vi "Cal Step.vi"(5 "Count":u8, 6 "DAC":u16[](array[numeric]), 7 "Gas Tank":u8, 9 "CalStatus":T1(ring), 10 "output cluster":T10, 11 "output cluster 3":T2 {"Current Settings"."Pump" items=["Pump 0", "Pump 1", "Pump 2", "Pump 3", "Pump 4", "Pump 5"]; "Current Settings"."Chart X axis Timescale" min=20 max=180 step=1; "Current Settings"."RunTime Mode Settings"."Exp. Gas Tank" items=["0.07", "0.031", "0.877", "1.863", "3.881", "5.790", "7.688", "6.000"]; "Current Settings"."RunTime Mode Settings"."Insp. Gas Tank" items=["0.07", "0.031", "0.877", "1.863", "3.881", "5.790", "7.688", "6.000"]; "Current Settings"."RunTime Mode Settings"."I:E Ratio" max=30 scale=0.0..7.0; "Current Settings"."RunTime Mode Settings"."Resp Rate Brpm" min=0 max=30 format="%.2f"; "Current Settings"."TE#2 Configuration"."Serial Port"."XOFF Char" format="%.0x"; "Current Settings"."TE#2 Configuration"."Serial Port"."XON Char" format="%.0x"; "Current Settings"."TE#2 Configuration"."Serial Port"."flow control" items=["None"=0, "XON/XOFF"=1, "RTS/CTS"=2, "DTR/DSR"=4]; "Current Settings"."TE#2 Configuration"."Serial Port"."stop bits" items=["1.0"=10, "1.5"=15, "2.0"=20]; "Current Settings"."TE#2 Configuration"."Serial Port"."data bits" min=5 max=8 step=1; "Current Settings"."TE#2 Configuration"."Serial Port"."baud rate" items=["75"=75, "110"=110, "134"=134, "150"=150, "300"=300, "600"=600, "1200"=1200, "1800"=1800, "2400"=2400, "4800"=4800, "7200"=7200, "9600"=9600, "14400"=14400, "19200"=19200, "28800"=28800, "38400"=38400, "56000"=56000, "57600"=57600, "115200"=115200, "128000"=128000, "230400"=230400]; "Current Settings"."TE#2 Configuration"."Serial Port"."termination char" format="%.0x"; "Current Settings"."TE#1 Configuration"."Serial Port"."XOFF Char" format="%.0x"; "Current Settings"."TE#1 Configuration"."Serial Port"."XON Char" format="%.0x"; "Current Settings"."TE#1 Configuration"."Serial Port"."flow control" items=["None"=0, "XON/XOFF"=1, "RTS/CTS"=2, "DTR/DSR"=4]; "Current Settings"."TE#1 Configuration"."Serial Port"."stop bits" items=["1.0"=10, "1.5"=15, "2.0"=20]; "Current Settings"."TE#1 Configuration"."Serial Port"."data bits" min=5 max=8 step=1; "Current Settings"."TE#1 Configuration"."Serial Port"."baud rate" items=["75"=75, "110"=110, "134"=134, "150"=150, "300"=300, "600"=600, "1200"=1200, "1800"=1800, "2400"=2400, "4800"=4800, "7200"=7200, "9600"=9600, "14400"=14400, "19200"=19200, "28800"=28800, "38400"=38400, "56000"=56000, "57600"=57600, "115200"=115200, "128000"=128000, "230400"=230400]; "Current Settings"."TE#1 Configuration"."Serial Port"."termination char" format="%.0x"; "Current Settings"."Capnometer Configuration"."Device" items=["None", "TidalWave", "LoFlow / Canary", "Capnogard"]; "Current Settings"."Capnometer Configuration"."Serial Port"."XOFF Char" format="%.0x"; "Current Settings"."Capnometer Configuration"."Serial Port"."XON Char" format="%.0x"; "Current Settings"."Capnometer Configuration"."Serial Port"."flow control" items=["None"=0, "XON/XOFF"=1, "RTS/CTS"=2, "DTR/DSR"=4]; "Current Settings"."Capnometer Configuration"."Serial Port"."stop bits" items=["1.0"=10, "1.5"=15, "2.0"=20]; "Current Settings"."Capnometer Configuration"."Serial Port"."data bits" min=5 max=8 step=1; "Current Settings"."Capnometer Configuration"."Serial Port"."baud rate" items=["75"=75, "110"=110, "134"=134, "150"=150, "300"=300, "600"=600, "1200"=1200, "1800"=1800, "2400"=2400, "4800"=4800, "7200"=7200, "9600"=9600, "14400"=14400, "19200"=19200, "28800"=28800, "38400"=38400, "56000"=56000, "57600"=57600, "115200"=115200, "128000"=128000, "230400"=230400]; "Current Settings"."Capnometer Configuration"."Serial Port"."termination char" format="%.0x"; "Current Settings"."DAQx Settings"."Analog Output Settings (Volts)" format="%#.3g"; "Current Settings"."DAQx Settings"."Duty Cycle" min=10.0 max=90.0 format="%.1g"; "Current Settings"."DAQx Settings"."Frequency" min=20.0 max=200.0; "Current Settings"."DataLogging Settings"."Data File Duration (Minutes)" min=2 max=200 format="%#.2g"; "Current Settings"."Calibration Settings"."Tolerance #2" min=2 max=4096; "Current Settings"."Calibration Settings"."Cal. Average" min=2 max=4096; "Current Settings"."Test Settings"."Test Sensor ID" items=["(select)", "RB", "YC", "", "Other"]}) -> (1 "NewCalStatus":T1(ring), 2 "New Count":u8)   [LabVIEW 2016]
uses:
  Controls/Cal Refs.ctl
  Controls/DAQ Needed.ctl
  Controls/Processed Variables.ctl
  Controls/AirPump Controls.ctl
  Controls/IE Ratio knob.ctl
  Controls/UI Settings.ctl
  Controls/Aux CO2 Control.ctl
  Controls/Serial Visa Control.ctl
  Controls/Aux CO2 Selector.ctl
  Controls/Aux TE Control.ctl
  Controls/Queues And Others.ctl
  <vilib>/Analysis/baseanly.llb/Mean (DBL).vi
  Miscellaneous/Globals.vi
  <vilib>/Analysis/NI_AALBase.lvlib
panel:
  # "Note: Setting Brpm to zero will\ndisable Insp / Exp digital output."
  # "mmHg"
  # "pts"
  # "tolerance"
  # "AN5 (Temp 1)"
  # "AN6 (Temp 2)"
  # "AN7 (Temp 3)"
  # "AN8 (T FET)"
  # "AN0 (T POT)"
  # "Tref (Set Pt))"
  # "(Spare)"
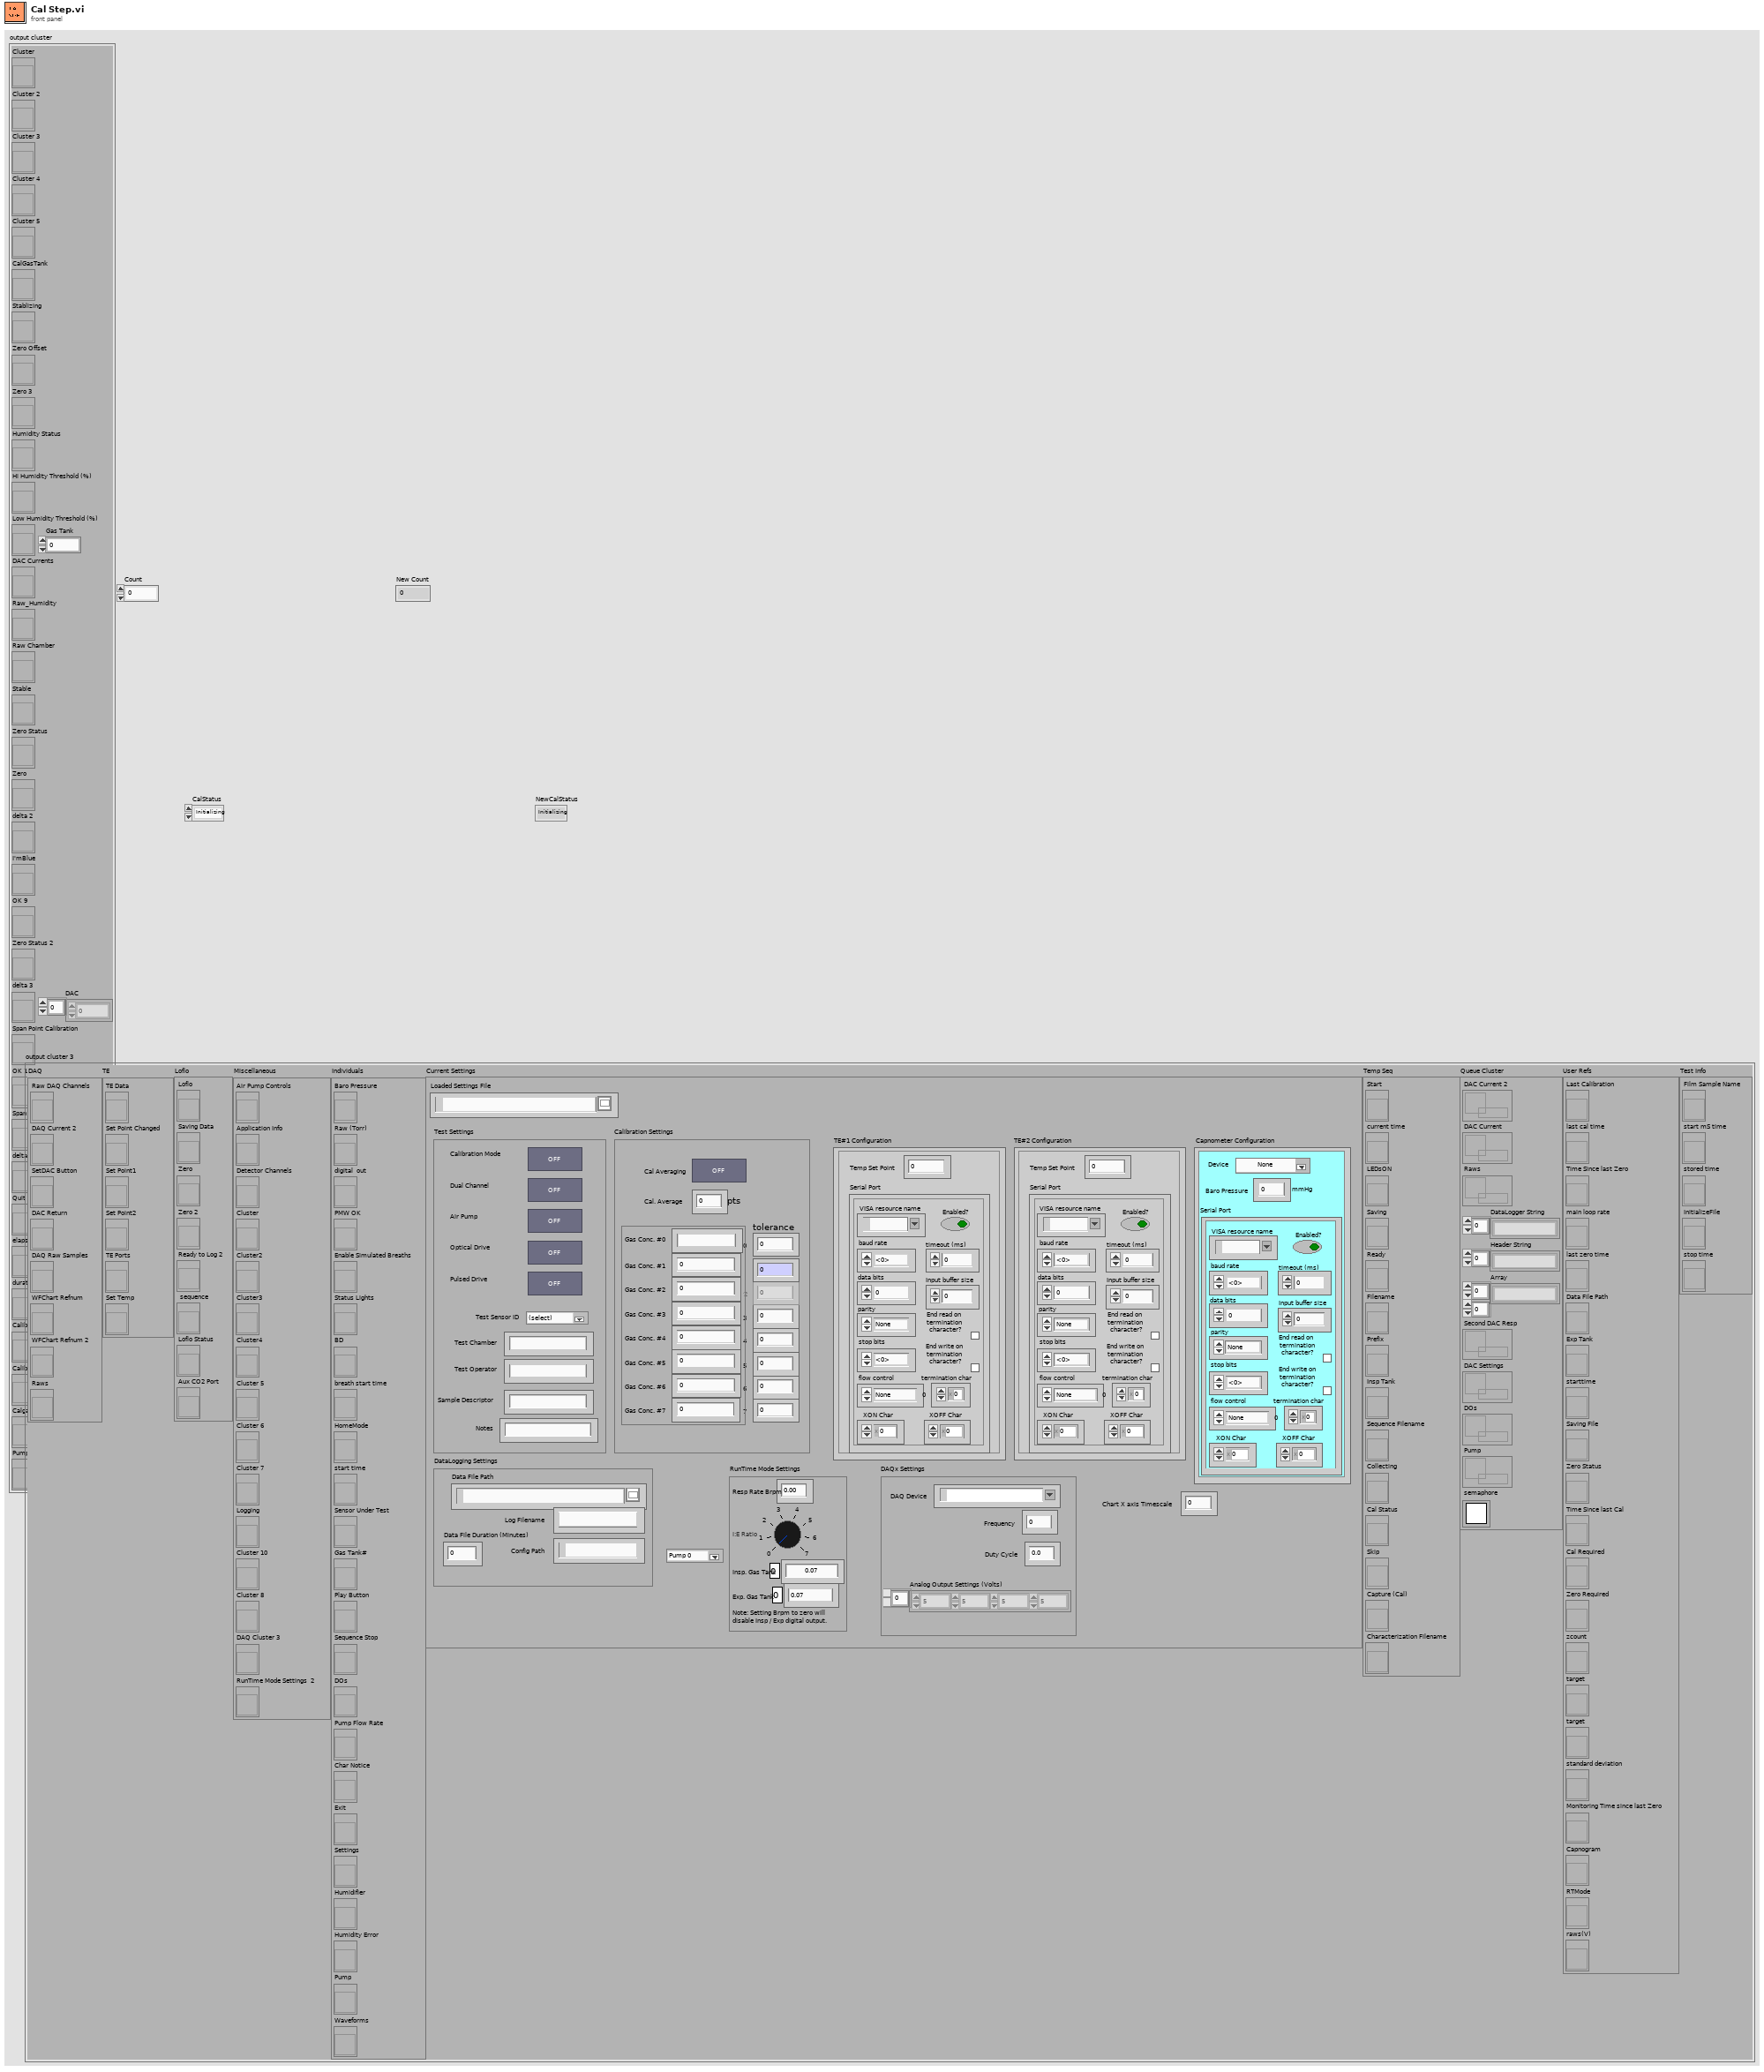
[diagram p1: front panel]
types:
  T1 = enum32{"Initializing", "Enter CO2 Value", "Enter Calibration Code", "Reading Calibration Data", "Stablizing", "Calculating Target Voltages", "Setting Zero Point", "Setting High Point", "Setting Span Point", "Calculating Gain & Offset", "Storing Calibration Coefficients", "Calibration Complete"}
  T2 = typedef "DAQ Needed.ctl" = cluster{"DAQ":cluster{"Raw DAQ Channels":refnum<vi>, "DAQ Current 2":refnum<vi>, "SetDAC Button":refnum<vi>, "DAC Return":refnum<vi>, "DAQ Raw Samples":refnum<vi>, "WFChart Refnum":refnum<vi>, "WFChart Refnum 2":refnum<vi>, "Raws":refnum<vi>}, "TE":cluster{"TE Data":refnum<vi>, "Set Point Changed":refnum<vi>, "Set Point1":refnum<vi>, "Set Point2":refnum<vi>, "TE Ports":refnum<vi>, "Set Temp":refnum<vi>}, "Loflo":cluster{"Loflo":refnum<vi>, "Saving Data":refnum<vi>, "Zero":refnum<vi>, "Zero 2":refnum<vi>, "Ready to Log 2":refnum<vi>, " sequence":refnum<vi>, "Loflo Status ":refnum<vi>, "Aux CO2 Port":refnum<vi>}, "Miscellaneous":cluster{"Air Pump Controls":refnum<vi>, "Application Info":refnum<vi>, "Detector Channels ":refnum<vi>, "Cluster":refnum<vi>, "Cluster2":refnum<vi>, "Cluster3":refnum<vi>, "Cluster4":refnum<vi>, "Cluster 5":refnum<vi>, "Cluster 6":refnum<vi>, "Cluster 7":refnum<vi>, "Logging":refnum<vi>, "Cluster 10":refnum<vi>, "Cluster 8":refnum<vi>, "DAQ Cluster 3":refnum<vi>, "RunTime Mode Settings  2":refnum<vi>}, "Individuals":cluster{"Baro Pressure":refnum<vi>, "Raw (Torr)":refnum<vi>, "digital  out":refnum<vi>, "PMW OK":refnum<vi>, "Enable Simulated Breaths":refnum<vi>, "Status Lights":refnum<vi>, "BD":refnum<vi>, "breath start time":refnum<vi>, "HomeMode":refnum<vi>, "start time":refnum<vi>, "Sensor Under Test":refnum<vi>, "Gas Tank#":refnum<vi>, "Play Button":refnum<vi>, "Sequence Stop":refnum<vi>, "DOs":refnum<vi>, "Pump Flow Rate":refnum<vi>, "Char Notice":refnum<vi>, "Exit":refnum<vi>, "Settings":refnum<vi>, "Humidifier":refnum<vi>, "Humidity Error":refnum<vi>, "Pump":refnum<vi>, "Waveforms":refnum<vi>}, "Current Settings":T3, "Temp Seq":cluster{"Start":refnum<vi>, "current time":refnum<vi>, "LEDsON":refnum<vi>, "Saving":refnum<vi>, "Ready":refnum<vi>, "Filename":refnum<vi>, "Prefix":refnum<vi>, "Insp Tank":refnum<vi>, "Sequence Filename":refnum<vi>, "Collecting":refnum<vi>, "Cal Status":refnum<vi>, "Skip":refnum<vi>, "Capture (Cal)":refnum<vi>, "Characterization Filename":refnum<vi>}, "Queue Cluster":T8, "User Refs":cluster{"Last Calibration":refnum<vi>, "last cal time":refnum<vi>, "Time Since last Zero":refnum<vi>, "main loop rate":refnum<vi>, "last zero time":refnum<vi>, "Data File Path":refnum<vi>, "Exp Tank":refnum<vi>, "starttime":refnum<vi>, "Saving File":refnum<vi>, "Zero Status":refnum<vi>, "Time Since last Cal":refnum<vi>, "Cal Required":refnum<vi>, "Zero Required":refnum<vi>, "zcount":refnum<vi>, "target":refnum<vi>, "target":refnum<vi>, "standard deviation":refnum<vi>, "Monitoring Time since last Zero":refnum<vi>, "Capnogram":refnum<vi>, "RTMode":refnum<vi>, "raws(V)":refnum<vi>}, "Test Info":cluster{"Film Sample Name":refnum<vi>, "start mS time":refnum<vi>, "stored time":refnum<vi>, "InitializeFile":refnum<vi>, "stop time":refnum<vi>}}
  T3 = typedef "UI Settings.ctl" = cluster{"Loaded Settings File":path, "Test Settings":cluster{"Dual Channel":bool, "Air Pump":bool, "Optical Drive":bool, "Pulsed Drive":bool, "Calibration Mode":bool, "Test Sensor ID":u16, "Test Chamber":string, "Test Operator":string, "Sample Descriptor":string, "Notes":string}, "Calibration Settings":cluster{"Cal. Average":u16, "Cal Averaging":bool, "Tolerance #0":sgl, "Tolerance #7":sgl, "Tolerance #6":sgl, "Tolerance #5":sgl, "Tolerance #4":sgl, "Tolerance #3":sgl, "Tolerance #2":sgl, "Tolerance #1":sgl, "Gas Tank Settings":cluster{"Gas Conc. #0":string, "Gas Conc. #1":sgl, "Gas Conc. #2":sgl, "Gas Conc. #3":sgl, "Gas Conc. #4":sgl, "Gas Conc. #5":sgl, "Gas Conc. #6":sgl, "Gas Conc. #7":sgl}}, "DataLogging Settings":cluster{"Data File Path":path, "Data File Duration (Minutes)":sgl, "Log Filename":string, "Config Path":path}, "DAQx Settings":cluster{"DAQ Device":tag, "Frequency":dbl, "Duty Cycle":dbl, "Analog Output Settings (Volts)":sgl[]}, "Capnometer Configuration":T4, "TE#1 Configuration":T7, "TE#2 Configuration":T7, "RunTime Mode Settings ":cluster{"Resp Rate Brpm ":sgl, "I:E Ratio":u8, "Insp. Gas Tank":u16, "Exp. Gas Tank":u16}, "Chart X axis Timescale":u16, "Pump":u16}
  T4 = typedef "Aux CO2 Control.ctl" = cluster{"Serial Port":T5, "Baro Pressure":u32, "Device":T6}
  T5 = typedef "Serial Visa Control.ctl" = cluster{"termination char":u8, "End read on termination character?":bool, "Enabled?":bool, "VISA resource name":refnum<visa-resource-name>, "baud rate":u32, "data bits":u16, "parity":enum16{"None", "Odd", "Even", "Mark", "Space"}, "stop bits":u16, "flow control":u16, "timeout (ms)":u32, "Input buffer size":u32, "End write on termination character?":bool, "XON Char":u8, "XOFF Char":u8}
  T6 = typedef "Aux CO2 Selector.ctl" = u16
  T7 = typedef "Aux TE Control.ctl" = cluster{"Temp Set Point":sgl, "Serial Port":T5}
  T8 = typedef "Queues And Others.ctl" = cluster{"DAC Current 2":refnum<queue>, "DAC Current":refnum<queue>, "Raws":refnum<queue>, "DataLogger String":string[], "Header String":string[], "Array":string[][], "Second DAC Resp":refnum<queue>, "DAC Settings":refnum<queue>, "DOs":refnum<queue>, "Pump":refnum<queue>, "semaphore":T9}
  T9 = typedef "Semaphore RefNum" = refnum<k1>
  T10 = typedef "Cal Refs.ctl" = cluster{"Cluster":refnum<vi>, "Cluster 2":refnum<vi>, "Cluster 3":refnum<vi>, "Cluster 4":refnum<vi>, "Cluster 5":refnum<vi>, "CalGasTank":refnum<vi>, "Stablizing":refnum<vi>, "Zero Offset":refnum<vi>, "Zero 3":refnum<vi>, "Humidity Status":refnum<vi>, "Hi Humidity Threshold (%)":refnum<vi>, "Low Humidity Threshold (%)":refnum<vi>, "DAC Currents":refnum<vi>, "Raw_Humidity":refnum<vi>, "Raw Chamber":refnum<vi>, "Stable":refnum<vi>, "Zero Status":refnum<vi>, "Zero":refnum<vi>, "delta 2":refnum<vi>, "I'mBlue":refnum<vi>, "OK 9":refnum<vi>, "Zero Status 2":refnum<vi>, "delta 3":refnum<vi>, "Span Point Calibration":refnum<vi>, "OK 10":refnum<vi>, "Span Good":refnum<vi>, "delta":refnum<vi>, "Quit":refnum<vi>, "elapsed time":refnum<vi>, "duration":refnum<vi>, "Calibration Complete -":refnum<vi>, "Calibration Complete":refnum<vi>, "Calgas":refnum<vi>, "Pump Settings":refnum<vi>}
  T11 = cluster{"Tcal_Chamber":dbl, "Tcal_PCB":dbl, "Tcal_Film":dbl, "Tcal_Humidity":dbl, "Tcal_Det":dbl[], "Cal Gas":dbl, "Reference":dbl}
  T12 = cluster{"CalFile Selected":path, "TYPE":string, "DATE":string, "C0FC2V":dbl[], "C6FC2V":dbl[], "V_0d(target)":dbl[], "V_6d(target)":dbl[], "V_span(target)":dbl[], "CHANNEL":string[], "Status":bool[], "BlueLED 2":bool[], "C2V":u8[], "A":dbl[], "B":dbl[], "C":dbl[], "D":dbl[], "V2C":u8[], "A'":dbl[], "B'":dbl[], "C'":dbl[], "D'":dbl[]}
  T13 = cluster{"CHANNEL 2":string[], "BlueLED":bool[], "V_RA(5mA)":dbl[], "V_RA(15mA)":dbl[], "mI":dbl[], "DAC scale":dbl[]}
  T14 = cluster{"V_0d(ImA)\nActual":dbl[], "V_6d(ImA)\nActual":dbl[], "V_span(ImA)":dbl[], "V_0(adjust)\ncal offsets":dbl[], "V_span(adjust)":dbl[], "Gain(adjust)":dbl[]}
  T15 = typedef "Calibration Coefficients.ctl" = cluster{"CalFile Used":path, "TYPE":string, "DATE":string, "Humidity":sgl, "Chamber Temp":dbl, "CO2_calgas":dbl, "V_(RA,5mA)":dbl, "V_(RA,15mA)":dbl, "mI":dbl, "V_0d_ImA (actual)":dbl, "V_6d_ImA (actual)":dbl, "I_span":dbl, "DAC":u16, "A":dbl, "B":dbl, "C":dbl, "D":dbl, "V6d":dbl, "A'":dbl, "B'":dbl, "C'":dbl, "D'":dbl, "V0d":dbl, "CalDate":string, "CalTime":string, "duration":dbl, "Detector Channel":string, "a2":dbl, "a3":dbl, "a4":dbl, "a5":dbl, "b2":dbl, "c2":dbl, "b3":dbl, "c3":dbl, "b4":dbl, "c4":dbl, "b5":dbl, "c5":dbl, "a7":dbl, "a8":dbl, "a9":dbl, "a10":dbl, "b7":dbl, "b8":dbl, "b9":dbl, "b10":dbl, "c7":dbl, "c8":dbl, "c9":dbl, "c10":dbl, "cal_offs_adj":dbl, "cal_gain_adj":dbl, "C6d":dbl, "C0d":dbl, "Cal_currernt":dbl, "C2V":u16, "V2C":u16, "Zero Date":string, "Zero Time":string, "Number of Zeroes":u16, "V_(()d, average)":dbl, "V_offs ":dbl, "G_adj":dbl, "Pump Flow Rate":u16, "Zero Required? ":bool, "Calibrate Required?":bool, "cal_utc":dbl, "zero_utc":dbl, "Elapsed Time":dbl, "PCB":string, "m0":dbl, "b0":dbl}
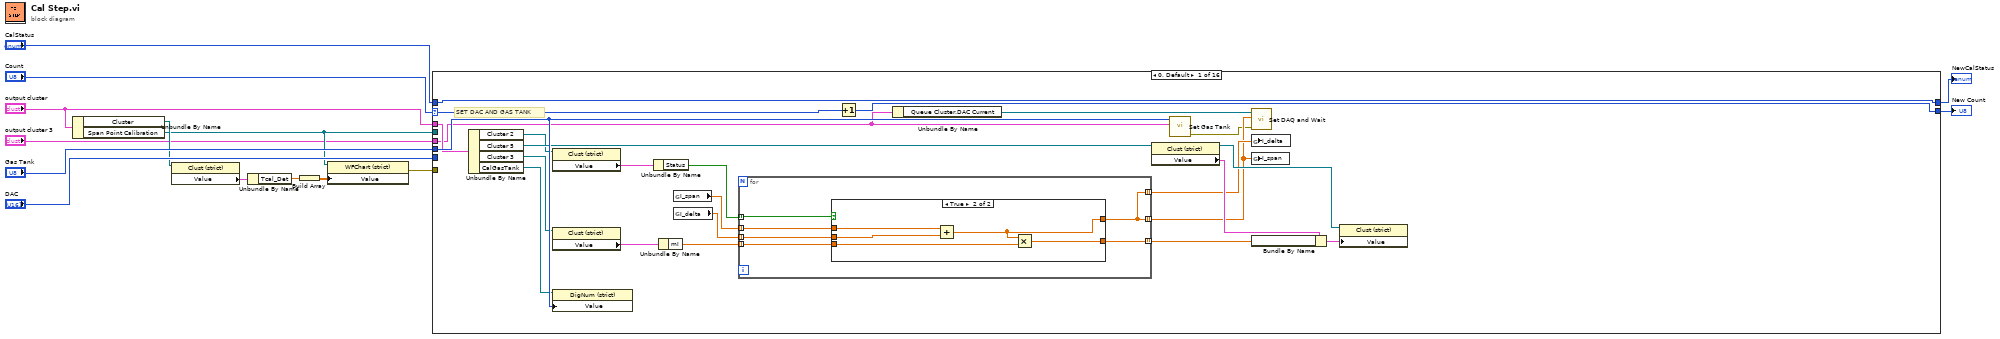
[diagram p0: block diagram]
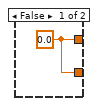
[diagram p2: hidden frame]
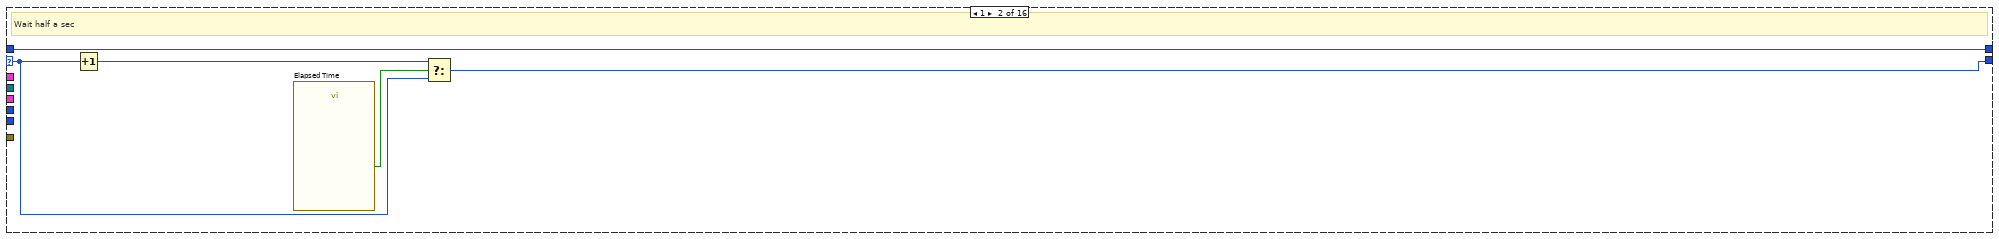
[diagram p3: hidden frame]
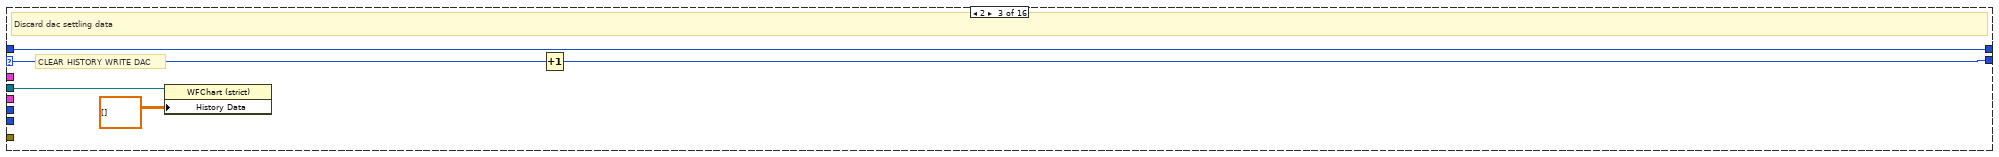
[diagram p4: hidden frame]
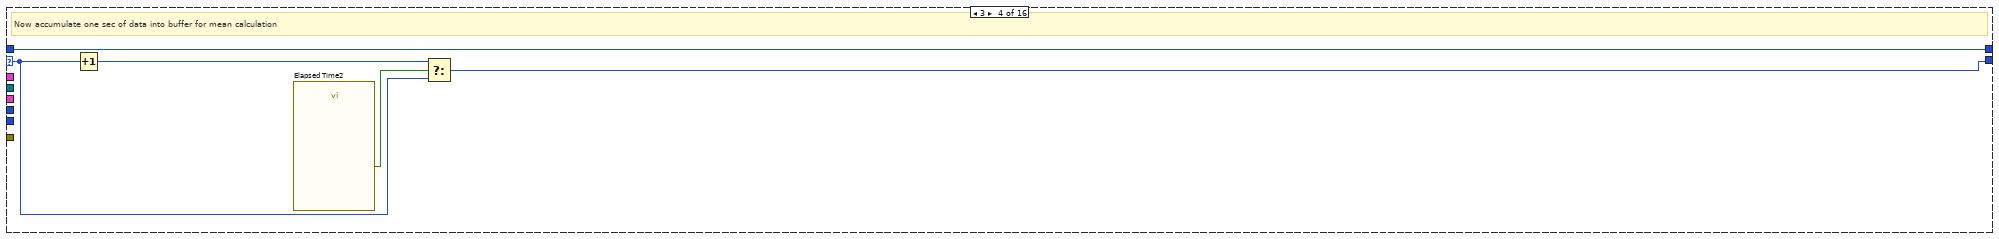
[diagram p5: hidden frame]
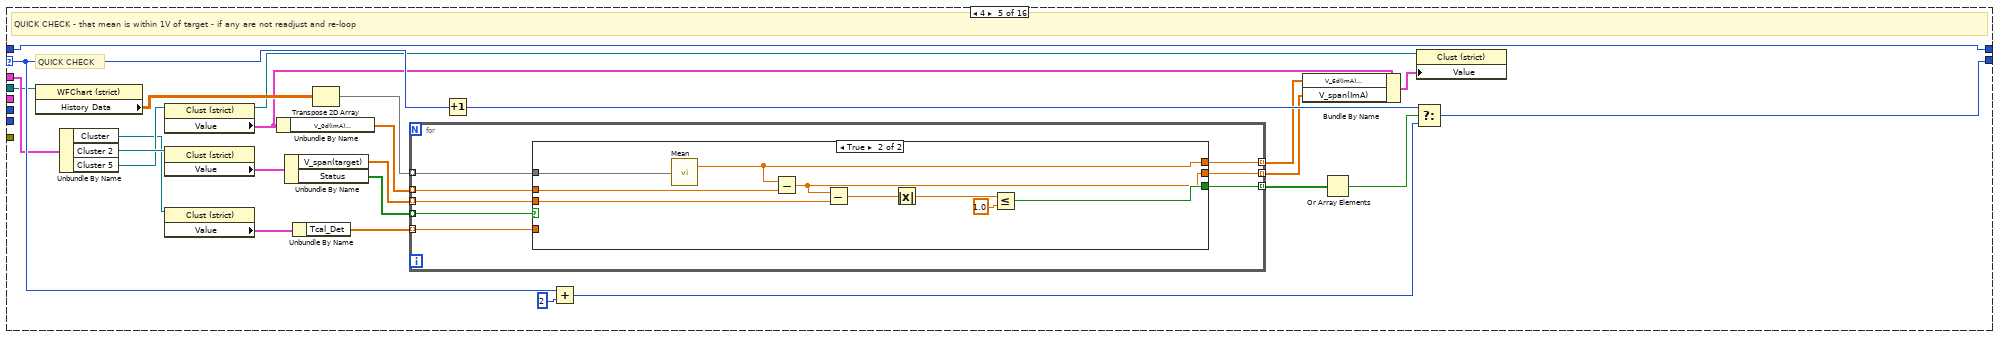
[diagram p6: hidden frame]
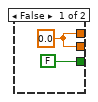
[diagram p7: hidden frame]
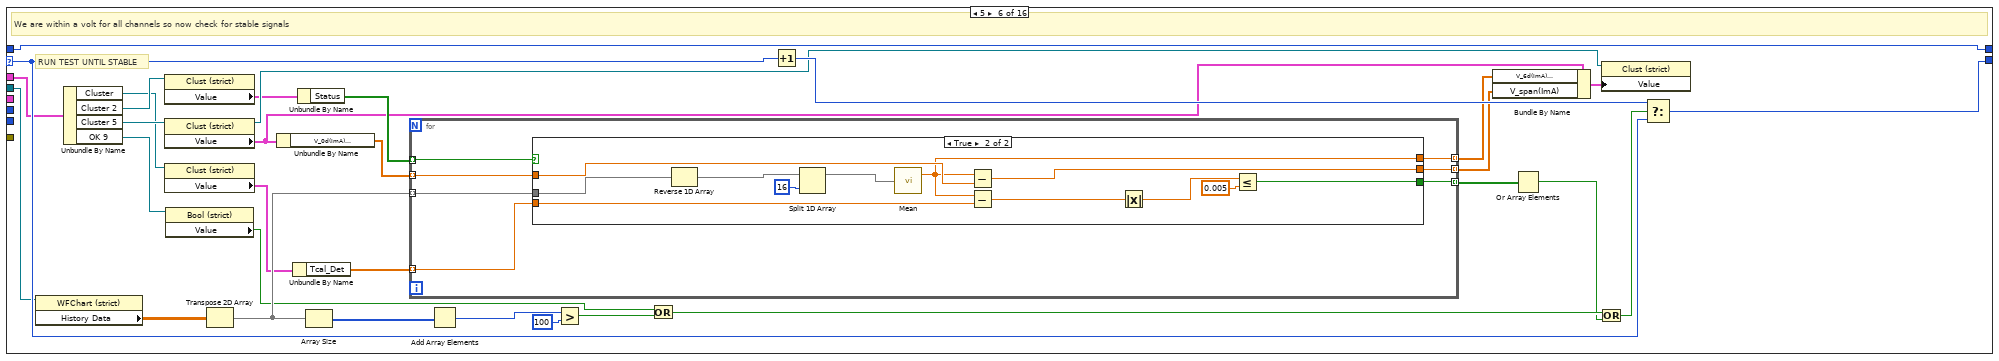
[diagram p8: hidden frame]
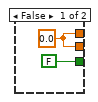
[diagram p9: hidden frame]
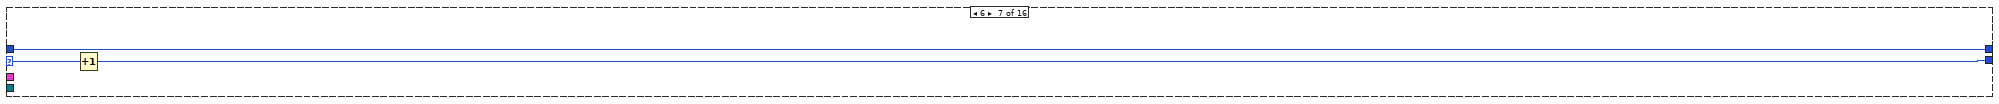
[diagram p10: hidden frame]
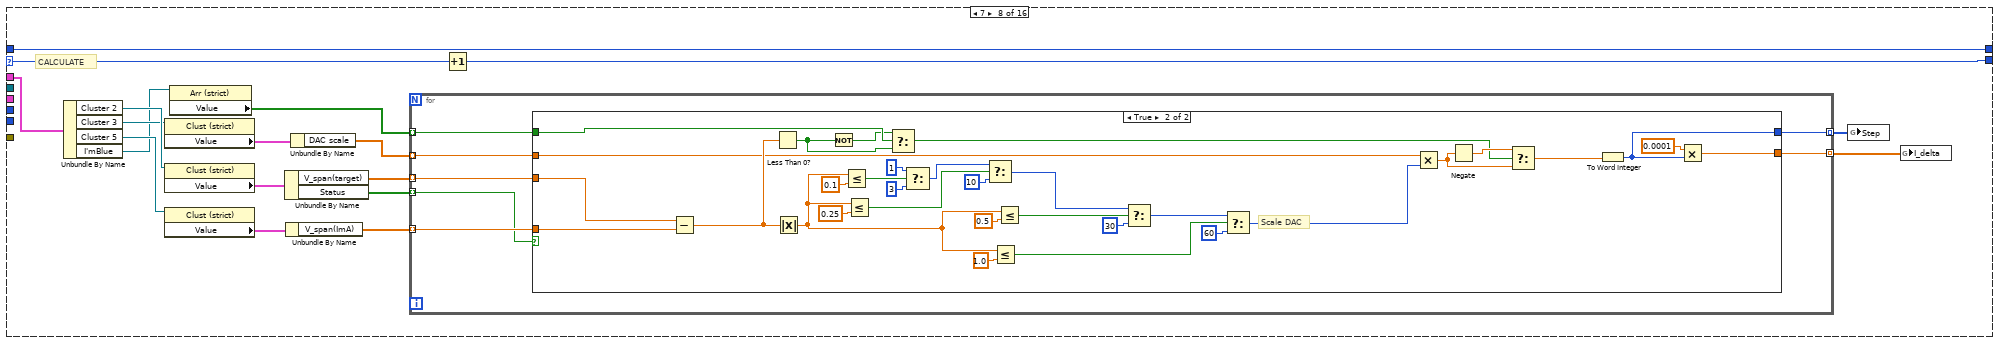
[diagram p11: hidden frame]
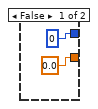
[diagram p12: hidden frame]
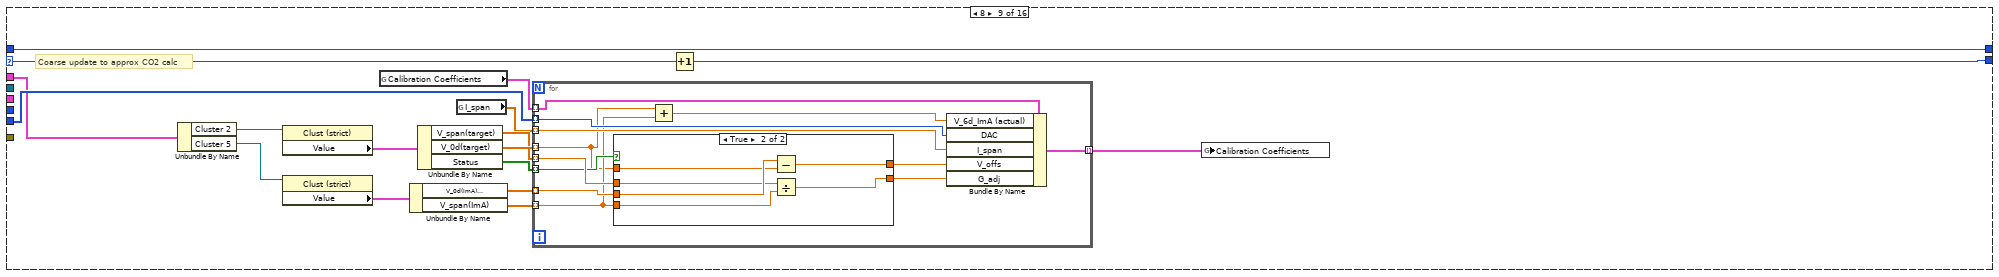
[diagram p13: hidden frame]
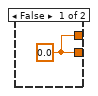
[diagram p14: hidden frame]
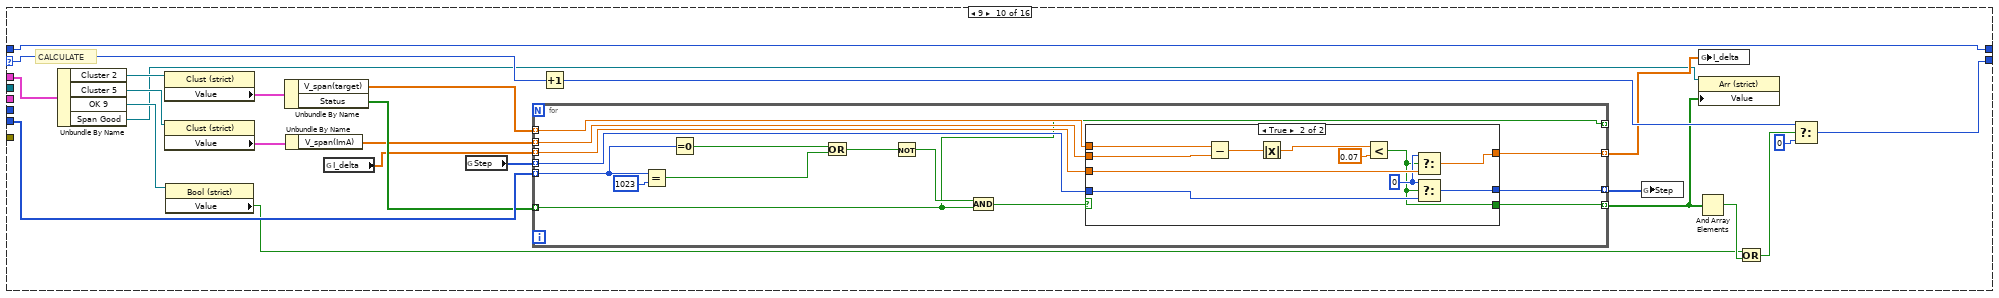
[diagram p15: hidden frame]
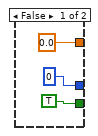
[diagram p16: hidden frame]
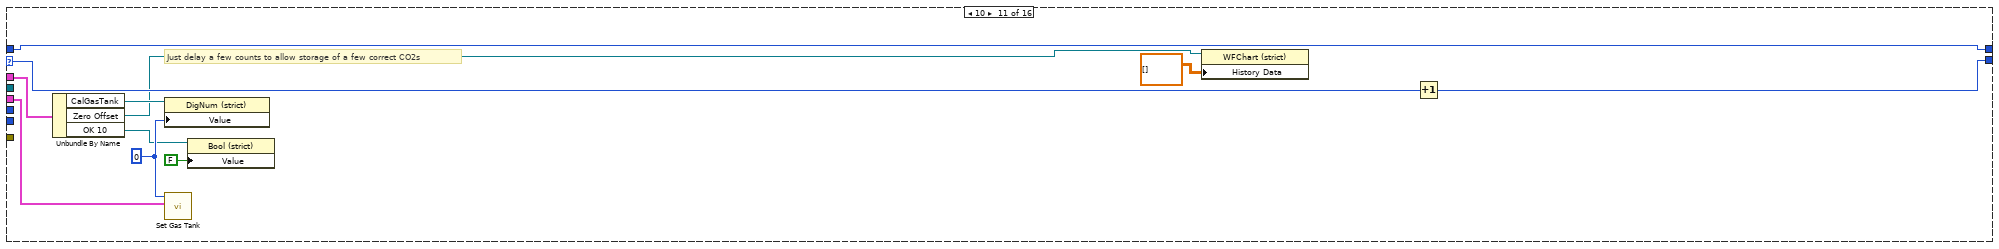
[diagram p17: hidden frame]
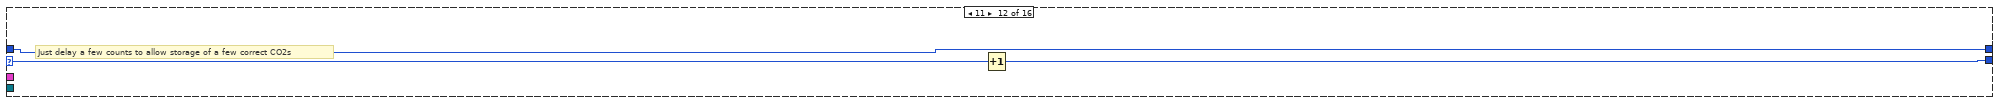
[diagram p18: hidden frame]
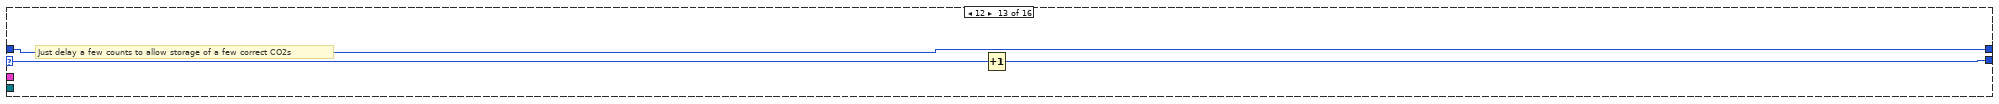
[diagram p19: hidden frame]
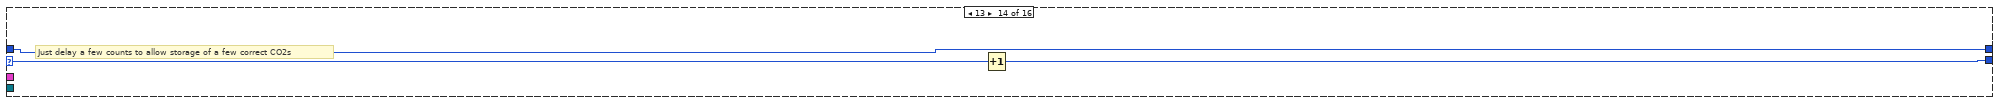
[diagram p20: hidden frame]
diagram:
  n1 = Unbundle By Name("output cluster") -> ("Cluster"=w9:refnum<vi>, "Span Point Calibration"=w6:refnum<vi>)
  n2 = property class="Clust (strict)"(reference=w9) -> ("Value"=w12:T11)  [unwired: 1 in, 2 out]
  n3 = Unbundle By Name(w12) -> ("Tcal_Det"=w11:dbl[])
  n4 = Build Array(w11) -> (w8:dbl[][])
  n5 = property class="WFChart (strict)"(reference=w6, "Value"=w8) -> (error out=w7:errorcluster)  [unwired: 1 in, 1 out]
  n6 = case shown="0, Default" "Count" {
    selector: "Count" -> [w37 w52 w60 w63 w88 w137 w165 w183 w241 w279 w324 w327 w330 w333 w336 _]
    tunnel: [w36 w54 w59 w62 w89 w138 w164 w181 w240 w280 w323 w326 w329 w332 w335 0 ("Step")] -> w1
    tunnel: "CalStatus" -> [w38 w55 w58 w65 w91 w141 w163 w182 w239 w284 w322 w325 w328 w331 w334 w339]
    tunnel: [w38 w55 w58 w65 w91 w141 w163 w182 w239 w284 w322 w325 w328 w331 w334 w337] -> w3
    tunnel: "Gas Tank" -> [w33 _ _ _ _ _ _ _ _ _ _ _ _ _ _ _]
    tunnel: "DAC" -> [_ _ _ _ _ _ _ _ w238 w276 _ _ _ _ _ _]
    tunnel: "output cluster 3" -> [w21 _ _ _ _ _ _ _ _ _ w315 _ _ _ _ _]
    tunnel: "output cluster" -> [w28 _ _ _ w77 w123 _ w180 w235 w274 w314 _ _ _ _ _]
    tunnel: w6 -> [_ _ w56 _ w66 w113 _ _ _ _ _ _ _ _ _ _]
    tunnel: w7 -> [_ _ _ _ _ _ _ _ _ _ _ _ _ _ _ _]
    frame 0, Default {
      # "SET DAC AND GAS TANK"
      n7 = Unbundle By Name(w28) -> ("Cluster 2"=w24:refnum<vi>, "Cluster 5"=w25:refnum<vi>, "Cluster 3"=w26:refnum<vi>, "CalGasTank"=w27:refnum<vi>)
      n8 = property class="Clust (strict)"(reference=w24) -> ("Value"=w23:T12)  [unwired: 1 in, 2 out]
      n9 = property class="Clust (strict)"(reference=w26) -> ("Value"=w35:T13)  [unwired: 1 in, 2 out]
      n10 = property class="DigNum (strict)"(reference=w27, "Value"=w33) -> ()  [unwired: 1 in, 2 out]
      n11 = Unbundle By Name(w23) -> ("Status"=w22:bool[])
      n12 = Unbundle By Name(w35) -> ("mI"=w34:dbl[])
      n13 = global read "Globals.vi" "I_span"() -> (w20:dbl[])
      n14 = global read "Globals.vi" "I_delta"() -> (w18:dbl[])
      n15 = for {
        tunnel: w34 -> [w42] mode=indexing
        tunnel: [w41] -> w29 mode=indexing
        tunnel: w20 -> [w44] mode=indexing
        tunnel: w18 -> [w43] mode=indexing
        tunnel: [w40] -> w19 mode=indexing
        tunnel: [w40] -> w16 mode=indexing
        tunnel: w22 -> [w39] mode=indexing
        n16 = case shown="True" w39 {
          tunnel: w44 -> [_ w50]
          tunnel: w43 -> [_ w49]
          tunnel: w42 -> [_ w48]
          tunnel: [w45 w47] -> w41
          tunnel: [w45 w46] -> w40
          frame False {
            w45 = 0.0
          }
          frame True {
            n17 = Add(x=w50, y=w49) -> (x+y=w46:dbl)
            n18 = Multiply(x=w46, y=w48) -> (x*y=w47:dbl)
          }
        }
      }
      n19 = Increment(x=w37) -> (x+1=w36:u8)
      n20 = Unbundle By Name(w21) -> ("Queue Cluster.DAC Current"=w17:refnum<queue>)
      n21 = property class="Clust (strict)"(reference=w25) -> (reference out=w32:refnum<vi>, "Value"=w31:T14)  [unwired: 1 in, 1 out]
      n22 = call "Set Gas Tank.vi"("input cluster"=w21, "Gas Tank"=w33) -> ("error out"=w15:errorcluster)  [unwired: 8 in, 1 out]
      n23 = call "Set DAQ and Wait.vi"("error in (no error)"=w15, "Array"=w16, "Queue in"=w17) -> ()  [unwired: 9 in]
      n24 = global write "Globals.vi" "I_delta"(w19) -> ()
      n25 = global write "Globals.vi" "I_span"(w16) -> ()
      n26 = Bundle By Name(cluster=w31, "V_0d(ImA)\nActual"=w29) -> (w30:T14)
      n27 = property class="Clust (strict)"(reference=w32, "Value"=w30) -> ()  [unwired: 1 in, 2 out]
    }
    frame 1 {
      # "Wait half a sec"
      n28 = Increment(x=w52) -> (x+1=w53:u8)
      n29 = call "Elapsed Time"() -> ("Time has Elapsed"=w51:bool)  [unwired: 12 in, 7 out]
      n30 = Select(t=w53, s=w51, f=w52) -> (s? t:f=w54:u8)
    }
    frame 2 {
      # "CLEAR HISTORY WRITE DAC"
      # "Discard dac settling data"
      n31 = property on="Property Node" class="WFChart (strict)"(reference=w56, "History Data"=dbl[][] []) -> ()  [unwired: 1 in, 2 out]
      n32 = Increment(x=w60) -> (x+1=w59:u8)
    }
    frame 3 {
      # "Now accumulate one sec of data into buffer for mean calculation"
      n33 = Increment(x=w63) -> (x+1=w64:u8)
      n34 = call "Elapsed Time2"() -> ("Time has Elapsed"=w61:bool)  [unwired: 12 in, 7 out]
      n35 = Select(t=w64, s=w61, f=w63) -> (s? t:f=w62:u8)
    }
    frame 4 {
      # "QUICK CHECK"
      # "QUICK CHECK - that mean is within 1V of target - if any are not readjust and re-loop"
      n36 = property on="Property Node" class="WFChart (strict)"(reference=w66) -> ("History Data"=w83:dbl[][])  [unwired: 1 in, 2 out]
      n37 = Unbundle By Name(w77) -> ("Cluster"=w71:refnum<vi>, "Cluster 2"=w76:refnum<vi>, "Cluster 5"=w73:refnum<vi>)
      n38 = property class="Clust (strict)"(reference=w73) -> (reference out=w81:refnum<vi>, "Value"=w68:T14)  [unwired: 1 in, 1 out]
      n39 = property class="Clust (strict)"(reference=w76) -> ("Value"=w75:T12)  [unwired: 1 in, 2 out]
      n40 = property class="Clust (strict)"(reference=w71) -> ("Value"=w72:T11)  [unwired: 1 in, 2 out]
      n41 = Unbundle By Name(w68) -> ("V_0d(ImA)\nActual"=w67:dbl[])
      n42 = Unbundle By Name(w75) -> ("V_span(target)"=w69:dbl[], "Status"=w74:bool[])
      n43 = Unbundle By Name(w72) -> ("Tcal_Det"=w70:dbl[])
      n44 = Transpose 2D Array(2D array=w83) -> (transposed array=w82:dbl[][])
      n45 = for {
        tunnel: w82 -> [w97] mode=indexing
        tunnel: [w99] -> w85 mode=indexing
        tunnel: w70 -> [w98] mode=indexing
        tunnel: [w95] -> w78 mode=indexing
        tunnel: [w96] -> w79 mode=indexing
        tunnel: w67 -> [w94] mode=indexing
        tunnel: w74 -> [w93] mode=indexing
        tunnel: w69 -> [w92] mode=indexing
        n46 = case shown="True" w93 {
          tunnel: [FALSE w110] -> w99
          tunnel: w98 -> [_ _]
          tunnel: w97 -> [_ w109]
          tunnel: [w101 w108] -> w96
          tunnel: [w101 w102] -> w95
          tunnel: w94 -> [_ w107]
          tunnel: w92 -> [_ w103]
          frame False {
            w101 = 0.0
          }
          frame True {
            n47 = call-poly <vilib>:"Mean.vi"("X"=w109) -> ("mean"=w108:dbl)  [unwired: 1 out]
            n48 = Subtract(x=w108, y=w107) -> (x-y=w102:dbl)
            n49 = Subtract(x=w102, y=w103) -> (x-y=w104:dbl)
            n50 = Absolute Value(x=w104) -> (abs(x)=w105:dbl)
            n51 = Less Or Equal?(x=w105, y=1.0) -> (x <= y?=w110:bool)
          }
        }
      }
      n52 = Increment(x=w88) -> (x+1=w90:u8)
      n53 = Add(x=w88, y=2) -> (x+y=w86:i32)
      n54 = Bundle By Name(cluster=w68, "V_6d(ImA)\nActual"=w79, "V_span(ImA)"=w78) -> (w80:T14)
      n55 = Or Array Elements(Boolean array=w85) -> (logical OR=w84:bool)
      n56 = Select(t=w90, s=w84, f=w86) -> (s? t:f=w89:i32)
      n57 = property class="Clust (strict)"(reference=w81, "Value"=w80) -> ()  [unwired: 1 in, 2 out]
    }
    frame 5 {
      # "RUN TEST UNTIL STABLE"
      # "We are within a volt for all channels so now check for stable signals"
      n58 = property on="Property Node" class="WFChart (strict)"(reference=w113) -> ("History Data"=w131:dbl[][])  [unwired: 1 in, 2 out]
      n59 = Unbundle By Name(w123) -> ("Cluster"=w117:refnum<vi>, "Cluster 2"=w122:refnum<vi>, "Cluster 5"=w119:refnum<vi>, "OK 9"=w112:refnum<vi>)
      n60 = property class="Clust (strict)"(reference=w122) -> ("Value"=w121:T12)  [unwired: 1 in, 2 out]
      n61 = property class="Clust (strict)"(reference=w119) -> (reference out=w127:refnum<vi>, "Value"=w115:T14)  [unwired: 1 in, 1 out]
      n62 = property class="Clust (strict)"(reference=w117) -> ("Value"=w118:T11)  [unwired: 1 in, 2 out]
      n63 = property class="Bool (strict)"(reference=w112) -> ("Value"=w111:bool)  [unwired: 1 in, 2 out]
      n64 = Transpose 2D Array(2D array=w131) -> (transposed array=w130:dbl[][])
      n65 = Unbundle By Name(w115) -> ("V_0d(ImA)\nActual"=w114:dbl[])
      n66 = Unbundle By Name(w118) -> ("Tcal_Det"=w116:dbl[])
      n67 = Unbundle By Name(w121) -> ("Status"=w120:bool[])
      n68 = Array Size(array=w130) -> (size(s)=w135:i32[])
      n69 = for {
        tunnel: w130 -> [w148] mode=indexing
        tunnel: [w147] -> w129 mode=indexing
        tunnel: w116 -> [w146] mode=indexing
        tunnel: [w145] -> w124 mode=indexing
        tunnel: [w144] -> w125 mode=indexing
        tunnel: w114 -> [w143] mode=indexing
        tunnel: w120 -> [w142] mode=indexing
        n70 = case shown="True" w142 {
          tunnel: w148 -> [_ w156]
          tunnel: [FALSE w155] -> w147
          tunnel: w146 -> [_ w154]
          tunnel: [w150 w153] -> w145
          tunnel: [w150 w151] -> w144
          tunnel: w143 -> [_ w152]
          frame False {
            w150 = 0.0 ("mean")
          }
          frame True {
            n71 = Reverse 1D Array(array=w156) -> (reversed array=w157:dbl[])
            n72 = Split 1D Array(array=w157, index=16) -> (first subarray=w158:dbl[])  [unwired: 1 out]
            n73 = call-poly <vilib>:"Mean.vi"("X"=w158) -> ("mean"=w151:dbl)  [unwired: 1 out]
            n74 = Subtract(x=w151, y=w152) -> (x-y=w153:dbl)
            n75 = Subtract(x=w151, y=w154) -> (x-y=w160:dbl)
            n76 = Absolute Value(x=w160) -> (abs(x)=w161:dbl)
            n77 = Less Or Equal?(x=w161, y=0.005) -> (x <= y?=w155:bool)
          }
        }
      }
      n78 = Add Array Elements(numeric array=w135) -> (sum=w132:i32)
      n79 = Greater?(x=w132, y=100 ("index")) -> (0:w134:bool)
      n80 = Or(x=w111, y=w134) -> (x .or. y?=w133:bool)
      n81 = Increment(x=w137) -> (x+1=w140:u8)
      n82 = Bundle By Name(cluster=w115, "V_6d(ImA)\nActual"=w125, "V_span(ImA)"=w124) -> (w126:T14)
      n83 = Or Array Elements(Boolean array=w129) -> (logical OR=w128:bool)
      n84 = Or(x=w133, y=w128) -> (x .or. y?=w139:bool)
      n85 = property class="Clust (strict)"(reference=w127, "Value"=w126) -> ()  [unwired: 1 in, 2 out]
      n86 = Select(t=w140, s=w139, f=w137) -> (s? t:f=w138:u8)
    }
    frame 6 {
      n87 = Increment(x=w165) -> (x+1=w164:u8)
    }
    frame 7 {
      # "CALCULATE"
      n88 = Unbundle By Name(w180) -> ("Cluster 2"=w179:refnum<vi>, "Cluster 3"=w176:refnum<vi>, "Cluster 5"=w171:refnum<vi>, "I'mBlue"=w167:refnum<vi>)
      n89 = property class="Clust (strict)"(reference=w176) -> ("Value"=w175:T13)  [unwired: 1 in, 2 out]
      n90 = property class="Clust (strict)"(reference=w179) -> ("Value"=w178:T12)  [unwired: 1 in, 2 out]
      n91 = property class="Clust (strict)"(reference=w171) -> ("Value"=w172:T14)  [unwired: 1 in, 2 out]
      n92 = property class="Arr (strict)"(reference=w167) -> ("Value"=w166:bool[])  [unwired: 1 in, 2 out]
      n93 = Unbundle By Name(w178) -> ("V_span(target)"=w173:dbl[], "Status"=w177:bool[])
      n94 = Unbundle By Name(w172) -> ("V_span(ImA)"=w170:dbl[])
      n95 = Unbundle By Name(w175) -> ("DAC scale"=w174:dbl[])
      n96 = for {
        tunnel: w173 -> [w188] mode=indexing
        tunnel: [w190] -> w169 mode=indexing
        tunnel: [w189] -> w168 mode=indexing
        tunnel: w170 -> [w187] mode=indexing
        tunnel: w177 -> [w186] mode=indexing
        tunnel: w166 -> [w185] mode=indexing
        tunnel: w174 -> [w184] mode=indexing
        n97 = case shown="True" w186 {
          tunnel: [0.0 w214] -> w190
          tunnel: [i8 0 ("t") w196] -> w189
          tunnel: w188 -> [_ w213]
          tunnel: w187 -> [_ w212]
          tunnel: w185 -> [_ w208]
          tunnel: w184 -> [_ w207]
          frame False {
          }
          frame True {
            # "Scale DAC"
            n98 = Subtract(x=w213, y=w212) -> (x-y=w219:dbl)
            n99 = Less Than 0?(x=w219) -> (x < 0?=w206:bool)
            n100 = Absolute Value(x=w219) -> (abs(x)=w201:dbl)
            n101 = Not(x=w206) -> (.not. x?=w205:bool)
            n102 = Less Or Equal?(x=w201, y=0.1) -> (x <= y?=w195:bool)
            n103 = Less Or Equal?(x=w201, y=0.25) -> (x <= y?=w220:bool)
            n104 = Select(t=w205, s=w208, f=w206) -> (s? t:f=w210:bool)
            n105 = Select(t=i8 1, s=w195, f=i8 3 ("t")) -> (s? t:f=w209:i8)
            n106 = Select(t=w209, s=w220, f=i8 10 ("t")) -> (s? t:f=w216:i8)
            n107 = Less Or Equal?(x=w201, y=1.0) -> (x <= y?=w202:bool)
            n108 = Less Or Equal?(x=w201, y=0.5) -> (x <= y?=w200:bool)
            n109 = Select(t=w216, s=w200, f=i8 30 ("t")) -> (s? t:f=w199:i8)
            n110 = Select(t=w199, s=w202, f=i8 60 ("t")) -> (s? t:f=w198:i8)
            n111 = Multiply(x=w207, y=w198) -> (x*y=w193:dbl)
            n112 = Negate(x=w193) -> (-x=w211:dbl)
            n113 = Select(t=w211, s=w210, f=w193) -> (s? t:f=w197:dbl)
            n114 = To Word Integer(number=w197) -> (16bit integer=w196:i16)
            n115 = Multiply(x=0.0001 ("y"), y=w196) -> (x*y=w214:dbl)
          }
        }
      }
      n116 = Increment(x=w183) -> (x+1=w181:u8)
      n117 = global write "Globals.vi" "Step"(w168) -> ()
      n118 = global write "Globals.vi" "I_delta"(w169) -> ()
    }
    frame 8 {
      # "Coarse update to approx CO2 calc"
      n119 = Unbundle By Name(w235) -> ("Cluster 2"=w234:refnum<vi>, "Cluster 5"=w231:refnum<vi>)
      n120 = property class="Clust (strict)"(reference=w234) -> ("Value"=w237:T12)  [unwired: 1 in, 2 out]
      n121 = property class="Clust (strict)"(reference=w231) -> ("Value"=w230:T14)  [unwired: 1 in, 2 out]
      n122 = global read "Globals.vi" "Calibration Coefficients"() -> (w226:T15[])
      n123 = Unbundle By Name(w230) -> ("V_0d(ImA)\nActual"=w229:dbl[], "V_span(ImA)"=w228:dbl[])
      n124 = Unbundle By Name(w237) -> ("V_span(target)"=w232:dbl[], "V_0d(target)"=w236:dbl[], "Status"=w233:bool[])
      n125 = global read "Globals.vi" "I_span"() -> (w227:dbl[])
      n126 = for {
        tunnel: w226 -> [w251] mode=indexing
        tunnel: [w250] -> w225 mode=indexing
        tunnel: w238 -> [w249] mode=indexing
        tunnel: w227 -> [w248] mode=indexing
        tunnel: w229 -> [w247] mode=indexing
        tunnel: w236 -> [w243] mode=indexing
        tunnel: w232 -> [w246] mode=indexing
        tunnel: w228 -> [w244] mode=indexing
        tunnel: w233 -> [w245] mode=indexing
        n127 = case shown="True" w245 {
          tunnel: [w254 w260] -> w253
          tunnel: [w254 w259] -> w252
          tunnel: w247 -> [_ w258]
          tunnel: w243 -> [_ w257]
          tunnel: w246 -> [_ w256]
          tunnel: w244 -> [_ w255]
          frame False {
            w254 = 0.0
          }
          frame True {
            n128 = Subtract(x=w258, y=w257) -> (x-y=w259:dbl)
            n129 = Divide(x=w256, y=w255) -> (x/y=w260:dbl)
          }
        }
        n130 = Add(x=w243, y=w244) -> (x+y=w242:dbl)
        n131 = Bundle By Name(cluster=w251, "V_6d_ImA (actual)"=w242, "DAC"=w249, "I_span"=w248, "V_offs"=w252, "G_adj"=w253) -> (w250:T15)
      }
      n132 = Increment(x=w241) -> (x+1=w240:u8)
      n133 = global write "Globals.vi" "Calibration Coefficients"(w225) -> ()
    }
    frame 9 {
      # "CALCULATE"
      n134 = Unbundle By Name(w274) -> ("Cluster 2"=w273:refnum<vi>, "Cluster 5"=w270:refnum<vi>, "OK 9"=w263:refnum<vi>, "Span Good"=w261:refnum<vi>)
      n135 = property class="Clust (strict)"(reference=w273) -> ("Value"=w275:T12)  [unwired: 1 in, 2 out]
      n136 = property class="Clust (strict)"(reference=w270) -> ("Value"=w269:T14)  [unwired: 1 in, 2 out]
      n137 = property class="Bool (strict)"(reference=w263) -> ("Value"=w262:bool)  [unwired: 1 in, 2 out]
      n138 = Unbundle By Name(w275) -> ("V_span(target)"=w271:dbl[], "Status"=w272:bool[])
      n139 = Unbundle By Name(w269) -> ("V_span(ImA)"=w268:dbl[])
      n140 = global read "Globals.vi" "I_delta"() -> (w266:dbl[])
      n141 = global read "Globals.vi" "Step"() -> (w264:i16[])
      n142 = for {
        tunnel: w271 -> [w299] mode=indexing
        tunnel: w268 -> [w298] mode=indexing
        tunnel: w264 -> [w297] mode=indexing
        tunnel: [w293] -> w277 mode=indexing
        tunnel: [w296] -> w265 mode=indexing
        tunnel: w266 -> [w295] mode=indexing
        tunnel: [w294] -> w267 mode=indexing
        tunnel: w276 -> [w289] mode=indexing
        tunnel: [w286] -> _ mode=indexing
        tunnel: w272 -> [w286] mode=indexing
        n143 = Equal?(x=w289, y=u16 1023) -> (x = y?=w291:bool)
        n144 = Equal To 0?(x=w289) -> (x = 0?=w292:bool)
        n145 = Or(x=w292, y=w291) -> (x .or. y?=w288:bool)
        n146 = Not(x=w288) -> (.not. x?=w287:bool)
        n147 = And(x=w287, y=w286) -> (x .and. y?=w285:bool)
        n148 = case shown="True" w285 {
          tunnel: w299 -> [_ w310]
          tunnel: w298 -> [_ w309]
          tunnel: w297 -> [_ w308]
          tunnel: [i8 0 ("Step") w307] -> w296
          tunnel: w295 -> [_ w306]
          tunnel: [0.0 ("V_(RA,5mA)") w304] -> w294
          tunnel: [TRUE w303] -> w293
          frame False {
          }
          frame True {
            w305 = i8 0 ("t")
            n149 = Subtract(x=w310, y=w309) -> (x-y=w311:dbl)
            n150 = Absolute Value(x=w311) -> (abs(x)=w312:dbl)
            n151 = Less?(x=w312, y=0.07) -> (x < y?=w303:bool)
            n152 = Select(t=w305, s=w303, f=w306) -> (s? t:f=w304:dbl)
            n153 = Select(t=w305, s=w303, f=w308) -> (s? t:f=w307:i16)
          }
        }
      }
      n154 = Increment(x=w279) -> (x+1=w282:u8)
      n155 = global write "Globals.vi" "Step"(w265) -> ()
      n156 = global write "Globals.vi" "I_delta"(w267) -> ()
      n157 = property class="Arr (strict)"(reference=w261, "Value"=w277) -> ()  [unwired: 1 in, 2 out]
      n158 = And Array Elements(Boolean array=w277) -> (logical AND=w278:bool)
      n159 = Or(x=w262, y=w278) -> (x .or. y?=w281:bool)
      n160 = Select(t=w282, s=w281, f=0) -> (s? t:f=w280:i32)
    }
    frame 10 {
      w319 = u8 0 ("CalGasTank")
      # "Just delay a few counts to allow storage of a few correct CO2s"
      n161 = Unbundle By Name(w314) -> ("CalGasTank"=w318:refnum<vi>, "Zero Offset"=w317:refnum<vi>, "OK 10"=w316:refnum<vi>)
      n162 = property class="DigNum (strict)"(reference=w318, "Value"=w319) -> ()  [unwired: 1 in, 2 out]
      n163 = call "Set Gas Tank.vi"("input cluster"=w315, "Gas Tank"=w319) -> ()  [unwired: 8 in, 2 out]
      n164 = property class="Bool (strict)"(reference=w316, "Value"=FALSE ("OK 10")) -> ()  [unwired: 1 in, 2 out]
      n165 = property on="Property Node" class="WFChart (strict)"(reference=w317, "History Data"=dbl[][] []) -> ()  [unwired: 1 in, 2 out]
      n166 = Increment(x=w324) -> (x+1=w323:u8)
    }
    frame 11 {
      # "Just delay a few counts to allow storage of a few correct CO2s"
      n167 = Increment(x=w327) -> (x+1=w326:u8)
    }
    frame 12 {
      # "Just delay a few counts to allow storage of a few correct CO2s"
      n168 = Increment(x=w330) -> (x+1=w329:u8)
    }
    frame 13 {
      # "Just delay a few counts to allow storage of a few correct CO2s"
      n169 = Increment(x=w333) -> (x+1=w332:u8)
    }
    frame 14 {
      # "Just delay a few counts to allow storage of a few correct CO2s"
      n170 = Increment(x=w336) -> (x+1=w335:u8)
    }
    frame 15 {
      # "Now Exit"
      n171 = Increment(x=w339) -> (x+1=w337:T1)
    }
  }
  "NewCalStatus" <- w3
  "New Count" <- w1
